vi "On New Frame Arrival.vi"(8 "error in (no error)":errorcluster, 10 "Control Ref":refnum<k24>, 11 "Camera_Prime95B in":refnum<class "Camera_Prime95B.lvclass">) -> (0 "error out":errorcluster, 3 "Camera_Prime95B out":refnum<class "Camera_Prime95B.lvclass">)   [LabVIEW 2020, in "Camera_Prime95B.lvlib" / "Camera_Prime95B.lvclass"]
uses:
  Camera_Prime95B.lvclass
  D:/Daguan/Development/MMicroscopyFramework/Model/Hardware Layer/Real Hardware/Camera_Prime95B/Camera_Prime95B/Dependencies/PVCamNET.dll
  Dependencies/PVCamNET.dll
  Controls/Camera Status.ctl
  Camera_Prime95B.lvclass/Camera_Prime95B.ctl
panel:
  out "BufferIndex":i32
  out "DroppedFrames":i32
  out "Fps":sgl
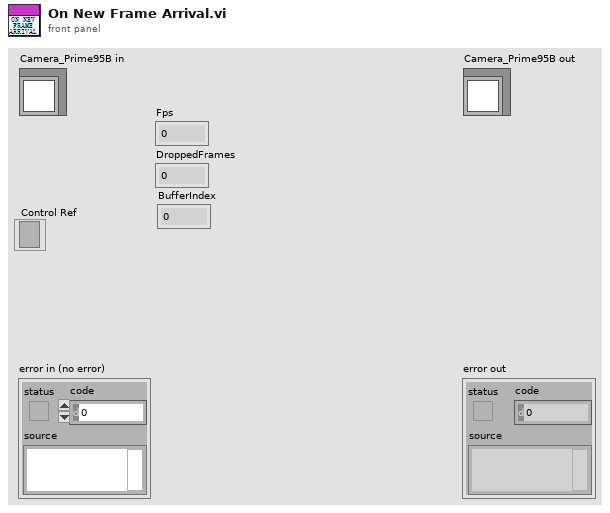
[diagram p1: front panel]
types:
  T1 = typedef "Camera_Prime95B.lvlib/Camera_Prime95B.lvclass/Camera Status.ctl" = i32
  T2 = typedef "IMAQ Image.ctl" = refnum<image>
  T3 = typedef "DataListener.lvclass/DataExchange.ctl" = cluster{"Source":string, "Destination":string, "Description":string, "value":variant}
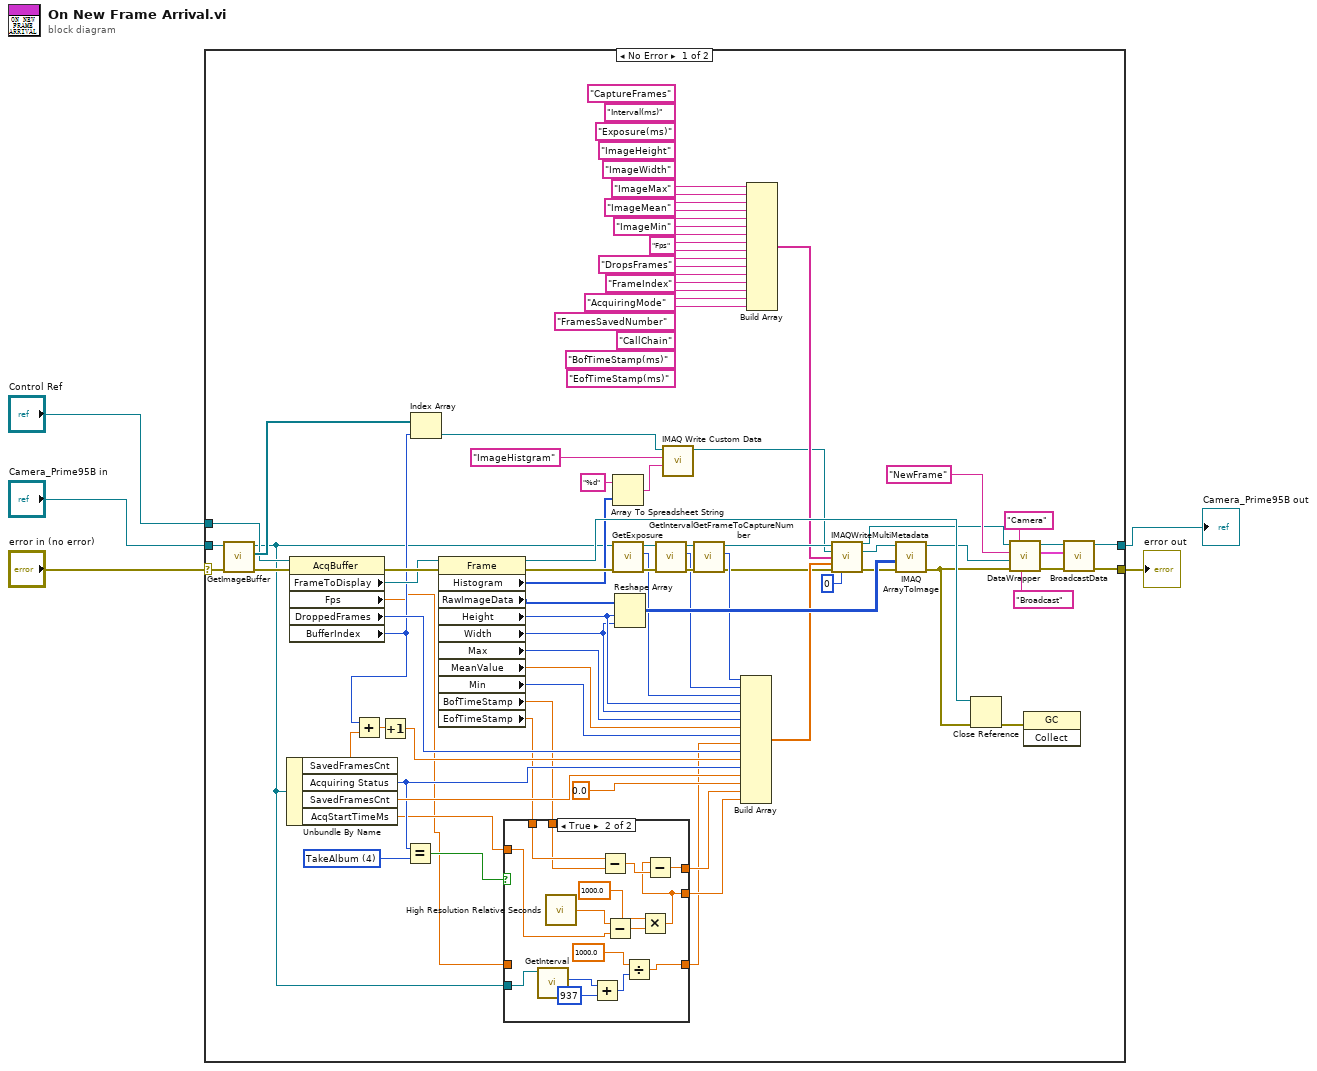
[diagram p0: block diagram]
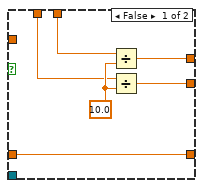
[diagram p2: hidden frame]
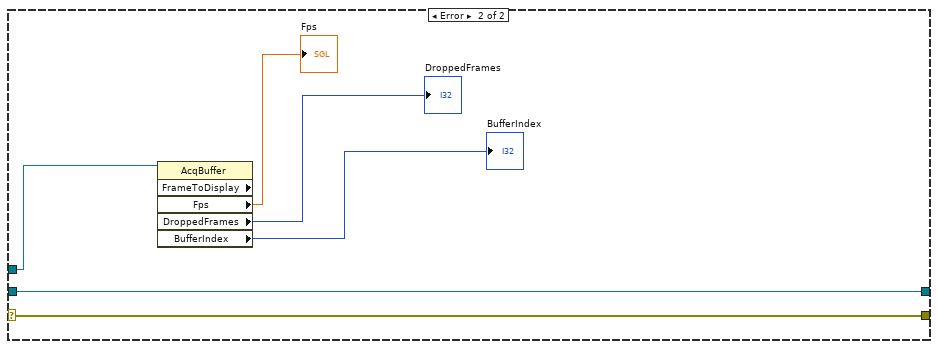
[diagram p3: hidden frame]
diagram:
  n1 = case shown="No Error" "error in (no error)" {
    selector: "error in (no error)" -> [w87 w113]
    tunnel: "Control Ref" -> [w81 w112]
    tunnel: "Camera_Prime95B in" -> [w86 w114]
    tunnel: [w29 w113] -> w2
    tunnel: [w27 w114] -> w1
    frame No Error {
      w18 = T1 4 items=["Idle", "Snap", "Live", "Capturing", "TakeAlbum"] ("y")
      n2 = call-dynamic "GetImageBuffer.vi"("error in (no error)"=w87, "Camera in"=w86) -> ("error out"=w80:errorcluster, "ImageBuffer"=w82:T2[], "Camera out"=w6:refnum<class "Camera_Prime95B.lvclass">)  [unwired: 6 in, 1 out]
      n3 = Unbundle By Name(w6) -> ("SavedFramesCnt"=w25:dbl, "Acquiring Status"=w17:T1, "SavedFramesCnt"=w19:dbl, "AcqStartTimeMs"=w9:dbl)
      n4 = property class="AcqBuffer"(reference=w81, error in=w80) -> (error out=w76:errorcluster, "FrameToDisplay"=w74:refnum<k24>, "Fps"=w8:sgl, "DroppedFrames"=w66:i32, "BufferIndex"=w24:i32)  [unwired: 1 out]
      n5 = Add(x=w24, y=w25) -> (x+y=w23:dbl)
      n6 = Increment(x=w23) -> (x+1=w22:dbl)
      n7 = Equal?(x=w17, y=w18) -> (x = y?=w16:bool)
      n8 = Index Array(array=w82, index=w24) -> (element=w43:T2)
      n9 = property class="Frame"(reference=w74, error in=w76) -> (reference out=w77:refnum<k24>, error out=w75:errorcluster, "Histogram"=w70:u32[], "RawImageData"=w71:i16[], "Height"=w73:u32, "Width"=w72:u32, "Max"=w69:u32, "MeanValue"=w68:dbl, "Min"=w67:u32, "BofTimeStamp"=w13:dbl, "EofTimeStamp"=w12:dbl)
      n10 = case shown="True" w16 {
        tunnel: w13 -> [w92 w105]
        tunnel: w12 -> [w91 w106]
        tunnel: [w90 w103] -> w11
        tunnel: [w89 w100] -> w10
        tunnel: w9 -> [_ w107]
        tunnel: w8 -> [w88 _]
        tunnel: [w88 w94] -> w7
        tunnel: w6 -> [_ w99]
        frame False {
          w93 = 10.0 ("y")
          n11 = Divide(x=w92, y=w93) -> (x/y=w90:dbl)
          n12 = Divide(x=w91, y=w93) -> (x/y=w89:dbl)
        }
        frame True {
          n13 = call-dynamic "GetInterval.vi"("Camera in"=w99) -> ("Setting.Interval"=w96:i32)  [unwired: 8 in, 2 out]
          n14 = call <vilib>:"High Resolution Relative Seconds.vi"() -> ("relative seconds"=w108:dbl)
          n15 = Add(x=w96, y=937) -> (x+y=w97:i32)
          n16 = Subtract(x=w106, y=w105) -> (x-y=w104:dbl)
          n17 = Subtract(x=w108, y=w107) -> (x-y=w102:dbl)
          n18 = Divide(x=1000.0, y=w97) -> (x/y=w94:dbl)
          n19 = Multiply(x=1000.0, y=w102) -> (x*y=w100:dbl)
          n20 = Subtract(x=w100, y=w104) -> (x-y=w103:dbl)
        }
      }
      n21 = Array To Spreadsheet String(array=w70, 3:"%d" ("format string")) -> (spreadsheet string=w42:string)  [unwired: 1 in]
      n22 = call-dynamic "GetExposure.vi"("error in (no error)"=w75, "Camera in"=w6) -> ("error out"=w57:errorcluster, "Setting.Exposure"=w52:i32, "Camera out"=w55:refnum<class "Camera_Prime95B.lvclass">)  [unwired: 7 in]
      n23 = Reshape Array(w71, w73, w72) -> (w79:i16[][])
      n24 = call-dynamic "GetInterval.vi"("error in (no error)"=w57, "Camera in"=w55) -> ("error out"=w56:errorcluster, "Setting.Interval"=w51:i32, "Camera out"=w54:refnum<class "Camera_Prime95B.lvclass">)  [unwired: 7 in]
      n25 = call "IMAQ Write Custom Data"("Custom Data In"=w42, "Key"="ImageHistgram", "Image"=w43) -> ("Image Out"=w40:T2)  [unwired: 7 in, 1 out]
      n26 = call-dynamic "GetFrameToCaptureNumber.vi"("error in (no error)"=w56, "Camera in"=w54) -> ("error out"=w30:errorcluster, "Setting.FramesToCapture"=w50:i32, "Camera out"=w53:refnum<class "Camera_Prime95B.lvclass">)  [unwired: 7 in]
      n27 = Build Array(w50, w51, w52, w73, w72, w69, w68, w67, w7, w66, w22, w17, w19, 0.0 ("element"), w11, w10) -> (w49:dbl[])
      n28 = Build Array("CaptureFrames" ("Key"), "Interval(ms)" ("Key"), "Exposure(ms)" ("Key"), "ImageHeight" ("Key"), "ImageWidth" ("Key"), "ImageMax" ("Key"), "ImageMean" ("Key"), "ImageMin" ("Key"), "Fps" ("Key"), "DropsFrames" ("Key"), "FrameIndex" ("Key"), "AcquiringMode" ("Key"), "FramesSavedNumber" ("Key"), "CallChain" ("element"), "BofTimeStamp(ms)" ("Key"), "EofTimeStamp(ms)" ("Key")) -> (w45:string[])
      n29 = call-dynamic "IMAQWriteMultiMetadata.vi"("GRMActor in"=w53, "Image In"=w40, "Keys"=w45, "Values"=w49, "error in (no error)"=w30, "precision (6)"=i16 0) -> ("GRMActor out"=w33:refnum<class "Camera_Prime95B.lvclass">, "Image Out"=w39:T2, "error out"=w44:errorcluster)  [unwired: 7 in]
      n30 = call "IMAQ ArrayToImage"("error in (no error)"=w44, "Image Pixels (I16)"=w79, "Image"=w39) -> ("error out"=w36:errorcluster, "Image Out"=w38:T2)  [unwired: 7 in]
      n31 = Close Reference(reference=w77, error in (no error)=w36) -> (error out=w37:errorcluster)
      n32 = call-dynamic "DataWrapper.vi"("Destination"="Broadcast" ("Type"), "Source"="Camera", "error in (no error)"=w36, "value"=w38, "Description"="NewFrame" ("Target"), "GRMActor in"=w33) -> ("error out"=w31:errorcluster, "DataExchange"=w26:T3, "GRMActor out"=w28:refnum<class "Camera_Prime95B.lvclass">)  [unwired: 3 in]
      n33 = invoke class="GC" method="Collect"(error in=w37) -> ()  [unwired: 2 in, 3 out]
      n34 = call-dynamic "BroadcastData.vi"("error in (no error)"=w31, "DataExchange"=w26, "GRMActor in"=w28) -> ("error out"=w29:errorcluster, "GRMActor out"=w27:refnum<class "Camera_Prime95B.lvclass">)  [unwired: 7 in]
    }
    frame Error {
      n35 = property class="AcqBuffer" props=["FrameToDisplay", "Fps", "DroppedFrames", "BufferIndex"](reference=w112) -> ("Fps"=→"Fps":sgl, "DroppedFrames"=→"DroppedFrames":i32, "BufferIndex"=→"BufferIndex":i32)  [unwired: 1 in, 3 out]
    }
  }
  "error out" <- w2
  "Camera_Prime95B out" <- w1
